vi "Get Relay State.vi"(8 "error in (no error)":errorcluster, 10 "SLSC Switch in":refnum<class "SLSC Switch.lvclass">, 11 "PhysicalChannelRelay in":refnum<class "PhysicalChannelRelay.lvclass">) -> (0 "error out":errorcluster, 1 "RelayPosition":T1=10 caption="position" items=["Open"=10, "Closed"=11], 2 "SLSC Switch out":refnum<class "SLSC Switch.lvclass">, 3 "PhysicalChannelRelay out":refnum<class "PhysicalChannelRelay.lvclass">)   [LabVIEW 2015, in "PhysicalChannelRelay.lvclass"]
uses:
  PhysicalChannelRelay.lvclass
  slscsl/RelayPosition.ctl
  SLSC Switch/SLSC Switch.lvclass
  SLSC Switch/SLSC Switch.lvclass/SLSC Switch.ctl
  PhysicalChannelRelay.lvclass/PhysicalChannelRelay.ctl
  <vilib>/SLSC/Get Phys Chan Property (Bool).vi
  slscsl/slscsl.lvclass
  <vilib>/SLSC/SLSC.lvlib
panel:
  out "property":refnum<k21>
  out "String":string
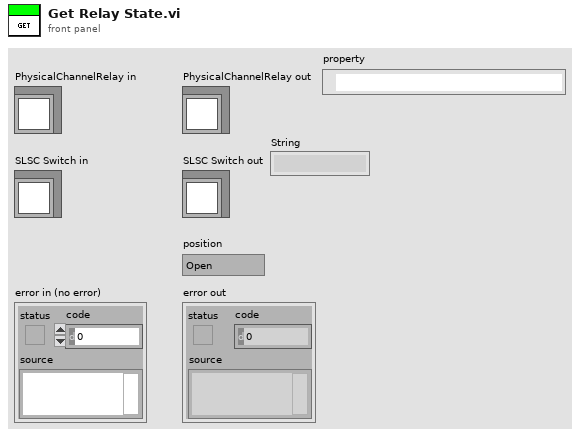
[diagram p1: front panel]
types:
  T1 = typedef "slscsl.lvclass/RelayPosition.ctl" = i32
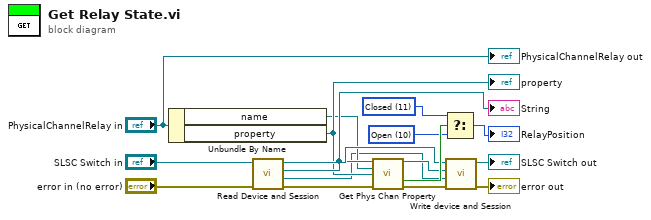
[diagram p0: block diagram]
diagram:
  w13 = T1 10 items=["Open"=10, "Closed"=11] ("f")
  w14 = T1 11 items=["Open"=10, "Closed"=11] ("RelayPosition")
  n1 = Unbundle By Name("PhysicalChannelRelay in") -> ("name"=w2:refnum<k21>, "property"=w3:refnum<k21>)
  "property" <- w3
  n2 = call "Read Device and Session.vi"("error in (no error)"="error in (no error)", "SLSC Switch in"="SLSC Switch in") -> ("error out"=w5:errorcluster, "device"=w1:refnum<k21>, "session"=w4:refnum<k21>, "SLSC Switch out"=w11:refnum<class "SLSC Switch.lvclass">)  [unwired: 6 in]
  "String" <- w4
  n3 = call-poly <vilib>:"Get Phys Chan Property.vi"("session in"=w4, "physical channels"=w2, "property"=w3, "error in (no error)"=w5) -> ("session out"=w10:refnum<k21>, "property value"=w15:bool, "error out"=w9:errorcluster)  [unwired: 9 in]
  n4 = Select(t=w14, s=w15, f=w13) -> (s? t:f=→"RelayPosition":T1)
  n5 = call "Write device and Session.vi"("error in (no error)"=w9, "device"=w1, "session"=w10, "SLSC Switch in"=w11) -> ("error out"=→"error out":errorcluster, "SLSC Switch out"=→"SLSC Switch out":refnum<class "SLSC Switch.lvclass">)  [unwired: 6 in]
  "PhysicalChannelRelay out" <- "PhysicalChannelRelay in"
